vi "getAndorCurrentTemperature.vi"(8 "error in (no error)":errorcluster, 11 "AndorIKonTempController.lvclass in":refnum<class "AndorIKonTempController.lvclass">) -> (0 "error out":errorcluster, 2 "currentTemperature":dbl, 3 "AndorIKonTempController.lvclass out":refnum<class "AndorIKonTempController.lvclass">)   [LabVIEW 2009, in "Hardware.lvlib" / "Channels.lvlib" / "AndorIKonTempController.lvclass"]
uses:
  AndorIKonTempController.lvclass
  AndorIKonTempController.lvclass/AndorIKonTempController.ctl
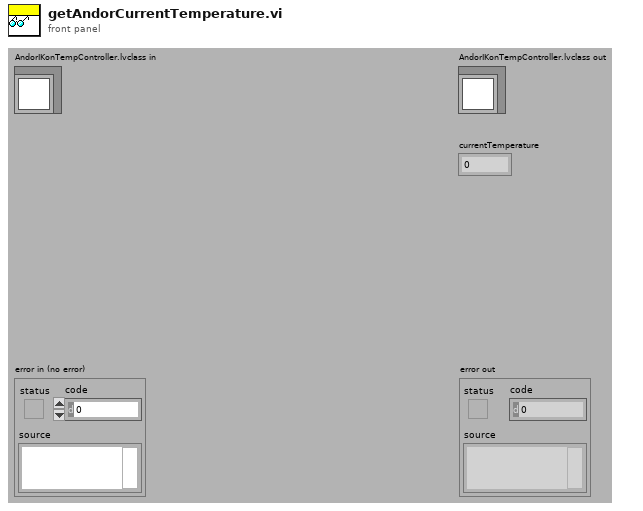
[diagram p1: front panel]
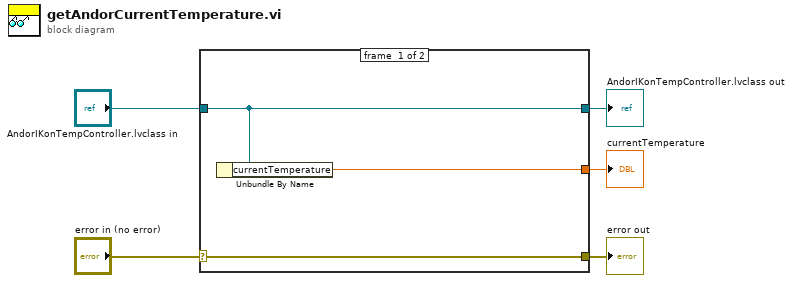
[diagram p0: block diagram]
diagram:
  n1 = case shown="No Error" "error in (no error)" {
    selector: "error in (no error)" -> [w8 w9]
    tunnel: [w8 w9] -> w4
    tunnel: [w7 w10] -> w2
    tunnel: "AndorIKonTempController.lvclass in" -> [w7 w10]
    tunnel: [w6 _] -> w1
    frame #0 {
      n2 = Unbundle By Name(w7) -> ("currentTemperature"=w6:dbl)
    }
    frame #1 {
    }
  }
  "error out" <- w4
  "AndorIKonTempController.lvclass out" <- w2
  "currentTemperature" <- w1
